vi "Init Notebook Rich Text Box.vi"(8 "Error In":errorcluster, 9 "Notebook Content":string, 11 ".NET Refnum in":refnum<k24>) -> (0 "Error Out":errorcluster)   [LabVIEW 2019, in "Notebook.lvlib"]
uses:
  Notebook.lvlib
  System.Windows.Forms
  System.Drawing
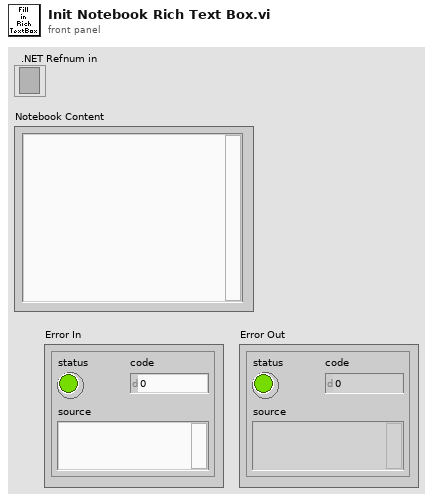
[diagram p1: front panel]
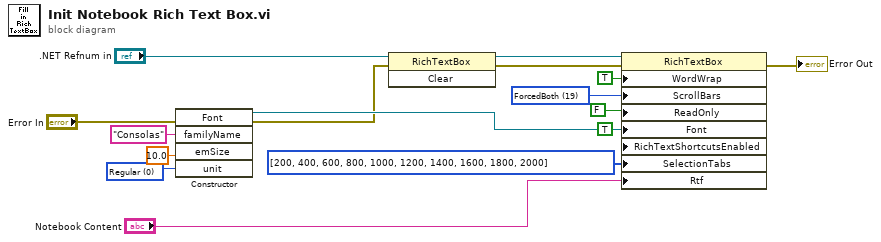
[diagram p0: block diagram]
diagram:
  w14 = 0 items=["Regular"=0, "Bold"=1, "Italic"=2, "Underline"=4, "Strikeout"=8] ("style")
  w5 = 19 items=["None"=0, "Horizontal"=1, "Vertical"=2, "Both"=3, "ForcedHorizontal"=17, "ForcedVertical"=18, "ForcedBoth"=19] ("ScrollBars")
  n1 = constructor class="Font"(error in="Error In", "familyName"="Consolas", "emSize"=sgl 10.0, "unit"=w14) -> (reference out=w16:refnum<k24>, error out=w8:errorcluster)  [unwired: 2 in, 4 out]
  n2 = invoke class="RichTextBox" method="Clear"(reference=".NET Refnum in", error in=w8) -> (reference out=w7:refnum<k24>, error out=w6:errorcluster)  [unwired: 1 in, 1 out]
  n3 = property class="RichTextBox"(reference=w7, error in=w6, "WordWrap"=TRUE, "ScrollBars"=w5, "ReadOnly"=FALSE ("Enabled"), "Font"=w16, "RichTextShortcutsEnabled"=TRUE, "SelectionTabs"=i32[] [200, 400, 600, 800, 1000, 1200, 1400, 1600, 1800, 2000], "Rtf"="Notebook Content") -> (error out=→"Error Out":errorcluster)  [unwired: 1 out]
